vi "Get Cancoder Absolute Angles.vi"(11 "Input Cancoders":T3) -> (0 "error out":errorcluster, 3 "offsets":cluster{dbl, dbl, dbl, dbl})   [LabVIEW 2020]
doc: "Get Cancoder Absolute Positions (Units are in Degrees)"
uses:
  <vilib>/Rock Robotics/WPI/ThirdParty/Phoenix-LabVIEW/CANCoder/Controls/CTRE_Phoenix_CANcoder_DeviceRef.ctl
  <vilib>/Rock Robotics/WPI/ThirdParty/Phoenix-LabVIEW/CANCoder/Get/CTRE_Phoenix_CANcoder_GetSensorData.vi
panel:
  out "cancoder current sensor pos":T1
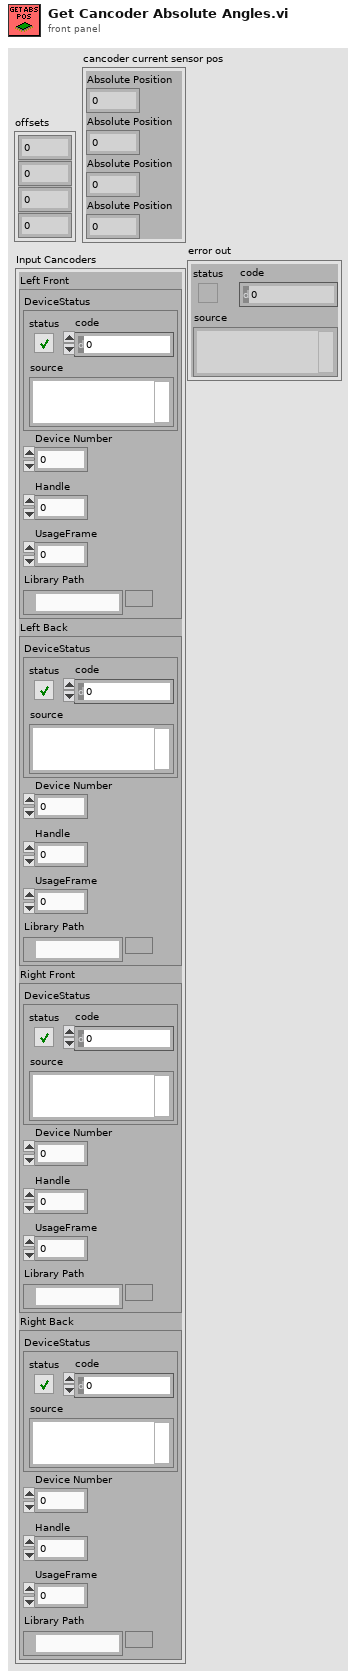
[diagram p1: front panel]
types:
  T1 = cluster{"Absolute Position":dbl, "Absolute Position":dbl, "Absolute Position":dbl, "Absolute Position":dbl}
  T2 = typedef "CTRE_Phoenix_CANcoder_DeviceRef.ctl" = cluster{"DeviceStatus":errorcluster, "Device Number":u8, "Handle":u64, "UsageFrame":u32, "Library Path":path}
  T3 = cluster{"Left Front":T2, "Left Back":T2, "Right Front":T2, "Right Back":T2}
  T4 = cluster{"LF (CC 9)":dbl, "LB (CC 10)":dbl, "RF (CC 11)":dbl, "RB (CC 12)":dbl}
  T5 = cluster{"angle out":dbl, "angle out":dbl, "angle out":dbl, "angle out":dbl}
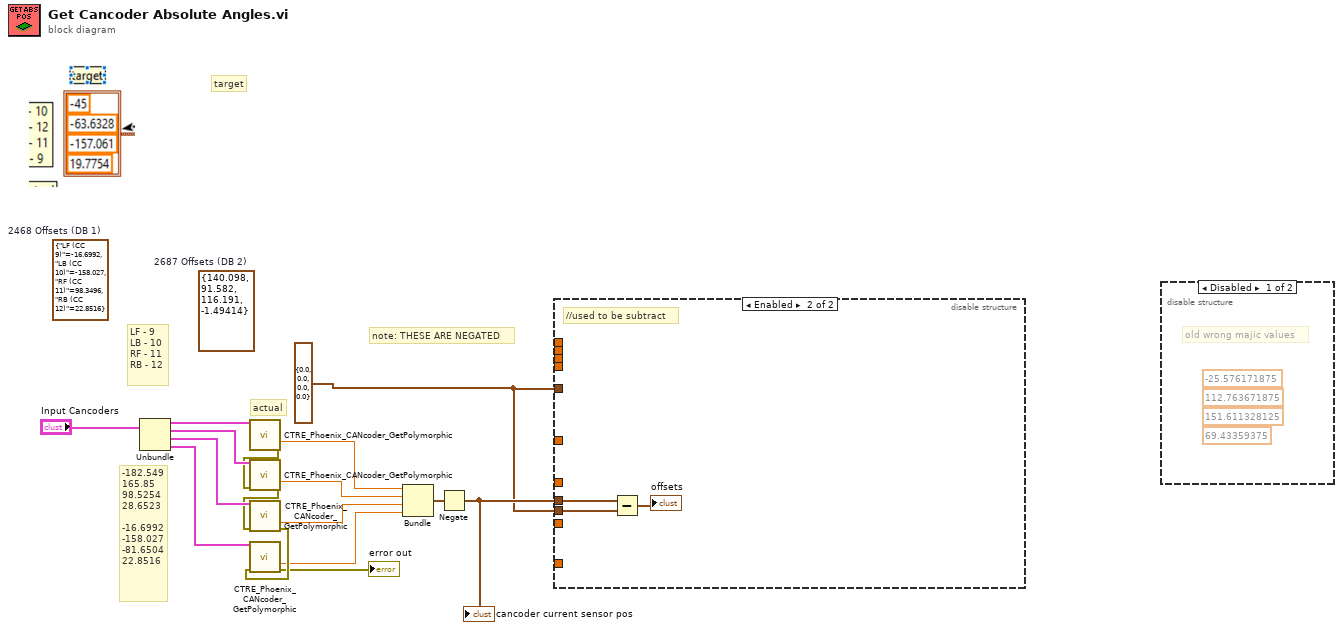
[diagram p0: block diagram]
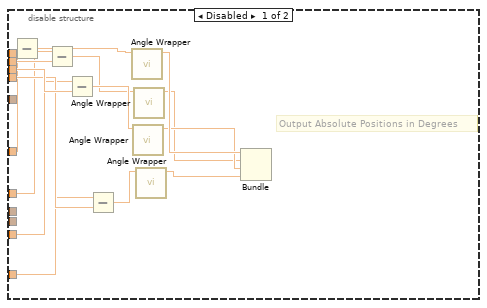
[diagram p3: hidden frame]
diagram:
  w2 = T1 {"Absolute Position"=0.0, "Absolute Position"=0.0, "Absolute Position"=0.0, "Absolute Position"=0.0}
  (unwired) T4 {"LF (CC 9)"=-16.6992, "LB (CC 10)"=-158.027, "RF (CC 11)"=98.3496, "RB (CC 12)"=22.8516}  # 2468 Offsets (DB 1)
  (unwired) T4 {"LF (CC 9)"=140.098, "LB (CC 10)"=91.582, "RF (CC 11)"=116.191, "RB (CC 12)"=-1.49414}  # 2687 Offsets (DB 2)
  # "-182.549\n165.85\n98.5254\n28.6523\n\n-16.6992\n-158.027\n-81.6504\n22.8516"
  # "note: THESE ARE NEGATED"
  # "target"
  # "actual"
  # "LF - 9 \nLB - 10\nRF - 11\nRB - 12"
  n1 = Unbundle("Input Cancoders") -> ("Left Front"=w15:T2, "Left Back"=w14:T2, "Right Front"=w13:T2, "Right Back"=w12:T2)
  n2 = call-poly <vilib>:"CTRE_Phoenix_CANcoder_GetPolymorphic.vi"("CTRE_CANcoder_DeviceRef"=w15) -> ("Absolute Position"=w8:dbl, "error out"=w11:errorcluster)  [unwired: 10 in, 3 out]
  n3 = call-poly <vilib>:"CTRE_Phoenix_CANcoder_GetPolymorphic.vi"("CTRE_CANcoder_DeviceRef"=w14, "error in"=w11) -> ("Absolute Position"=w7:dbl, "error out"=w10:errorcluster)  [unwired: 9 in, 3 out]
  n4 = call-poly <vilib>:"CTRE_Phoenix_CANcoder_GetPolymorphic.vi"("CTRE_CANcoder_DeviceRef"=w13, "error in"=w10) -> ("Absolute Position"=w6:dbl, "error out"=w9:errorcluster)  [unwired: 9 in, 3 out]
  n5 = call-poly <vilib>:"CTRE_Phoenix_CANcoder_GetPolymorphic.vi"("CTRE_CANcoder_DeviceRef"=w12, "error in"=w9) -> ("Absolute Position"=w5:dbl, "error out"=→"error out":errorcluster)  [unwired: 9 in, 3 out]
  n6 = Bundle("Absolute Position"=w8, "Absolute Position"=w7, "Absolute Position"=w6, "Absolute Position"=w5) -> (w4:T1)  [unwired: 1 in]
  n7 = Negate(x=w4) -> (-x=w3:T1)
  "cancoder current sensor pos" <- w3
  n8 = disable-structure shown="Enabled" {
    disable-tunnel: _ -> [w33 _]
    disable-tunnel: _ -> [w32 _]
    disable-tunnel: _ -> [w31 _]
    disable-tunnel: _ -> [w30 _]
    disable-tunnel: _ -> [w20 _]
    disable-tunnel: _ -> [w19 _]
    disable-tunnel: _ -> [w18 _]
    disable-tunnel: _ -> [w17 _]
    disable-tunnel: w3 -> [_ w34]
    disable-tunnel: w2 -> [_ w36]
    disable-tunnel: w2 -> [_ _]
    frame Disabled {
      # "Output Absolute Positions in Degrees"
      n9 = Subtract(x=w20, y=w33) -> (x-y=w28:dbl)
      n10 = Subtract(x=w19, y=w32) -> (x-y=w24:dbl)
      n11 = Subtract(x=w18, y=w31) -> (x-y=w26:dbl)
      n12 = Subtract(x=w17, y=w30) -> (x-y=w22:dbl)
      n13 = call "Angle Wrapper.vi"("angle in"=w28) -> ("angle out"=w27:dbl)  [unwired: 10 in]
      n14 = call "Angle Wrapper.vi"("angle in"=w26) -> ("angle out"=w25:dbl)  [unwired: 10 in]
      n15 = call "Angle Wrapper.vi"("angle in"=w24) -> ("angle out"=w23:dbl)  [unwired: 10 in]
      n16 = call "Angle Wrapper.vi"("angle in"=w22) -> ("angle out"=w21:dbl)  [unwired: 10 in]
      n17 = Bundle("angle out"=w27, "angle out"=w23, "angle out"=w25, "angle out"=w21) -> (w29:T5)  [unwired: 1 in]
    }
    frame Enabled {
      # "//used to be subtract"
      n18 = Subtract(x=w34, y=w36) -> (x-y=→"offsets":T1)
    }
  }
  n19 = disable-structure shown="Disabled" {
    frame Disabled {
      (unwired) -25.576171875 ("Absolute Position")
      (unwired) 112.763671875 ("Absolute Position")
      (unwired) 151.611328125 ("Absolute Position")
      (unwired) 69.43359375 ("Absolute Position")
      # "old wrong majic values"
    }
    frame Enabled {
    }
  }
